vi "File Extension Found.vi"(8 "error in (no error)":errorcluster, 10 "patterns":string, 11 "lowercase file extension":string) -> (0 "error out":errorcluster, 1 "match?":bool, 2 "(lower case) pattern array":string[](array[string]), 3 "(lower case) extension array":string[](array[string]))   [LabVIEW 2021, in "Files.lvlib"]
uses:
  f3d61ee5-7587-452d-a064-bb003209bc5d.vi
  Files.lvlib
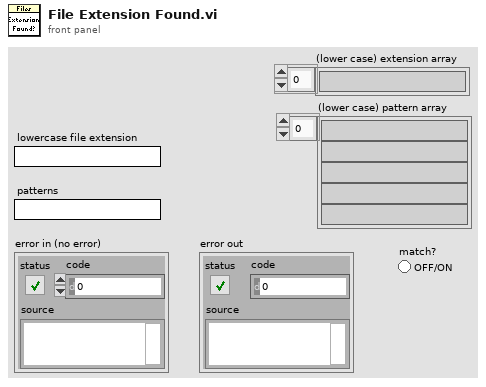
[diagram p1: front panel]
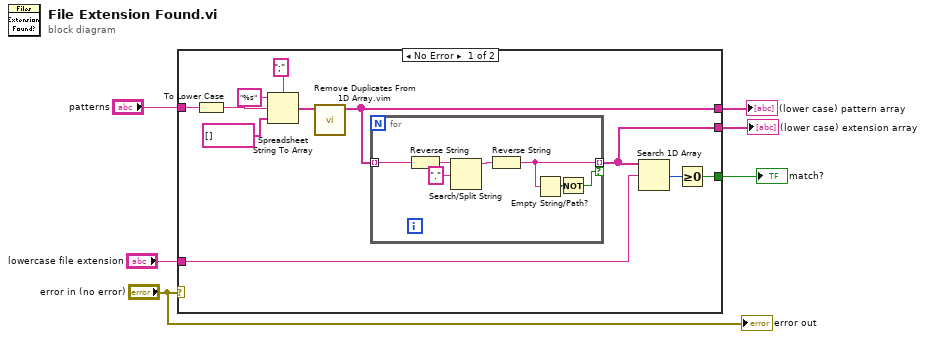
[diagram p0: block diagram]
diagram:
  n1 = case shown="No Error" "error in (no error)" {
    tunnel: "patterns" -> [w17 _]
    tunnel: [w7 _] -> w5
    tunnel: [w11 _] -> w4
    tunnel: "lowercase file extension" -> [w10 _]
    tunnel: [w8 _] -> w2
    frame No Error {
      n2 = To Lower Case(string=w17) -> (all lower case string=w13:string)
      n3 = Spreadsheet String To Array(delimiter (Tab)=";", format string="%s", spreadsheet string=w13, array type (2D Dbl)=string[] [] ("patterns")) -> (array=w12:string[])
      n4 = call "Remove Duplicates From 1D Array.vim"("array"=w12) -> ("array with duplicates removed"=w7:string[])  [unwired: 10 in]
      n5 = for {
        tunnel: w7 -> [w24] mode=indexing
        tunnel: [w20] -> w11 mode=indexing if=w18
        n6 = Reverse String(1:w24) -> (0:w23:string)
        n7 = Search/Split String(string=w23, search string/char (-)="." ("regular expression")) -> (substring before match=w21:string)  [unwired: 1 in, 2 out]
        n8 = Reverse String(1:w21) -> (0:w20:string)
        n9 = Empty String/Path?(string/path=w20) -> (empty?=w19:bool)
        n10 = Not(x=w19) -> (.not. x?=w18:bool)
      }
      n11 = Search 1D Array(1D array=w11, element=w10) -> (index of element=w9:i32)  [unwired: 1 in]
      n12 = Greater Or Equal To 0?(x=w9) -> (x >= 0?=w8:bool)
    }
    frame Error {
    }
  }
  "match?" <- w2
  "(lower case) pattern array" <- w5
  "(lower case) extension array" <- w4
  "error out" <- "error in (no error)"
